vi "导轨移动.vi"(0 "绝对位置":dbl, 1 "速度":i32, 5 "高温平板相对位置":dbl, 7 "低温平板相对位置":dbl, 11 "error in":errorcluster, 12 "移动至高温？":bool, 13 "默认位置":bool, 14 "执行程序零":bool) -> (8 "位置坐标":dbl, 15 "error IO":errorcluster)   [LabVIEW 2016]
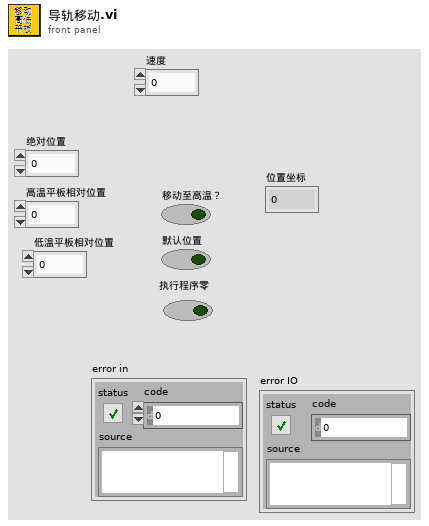
[diagram p1: front panel]
types:
  T1 = enum16{"read", "write", "release", "initial", "position calibration"}
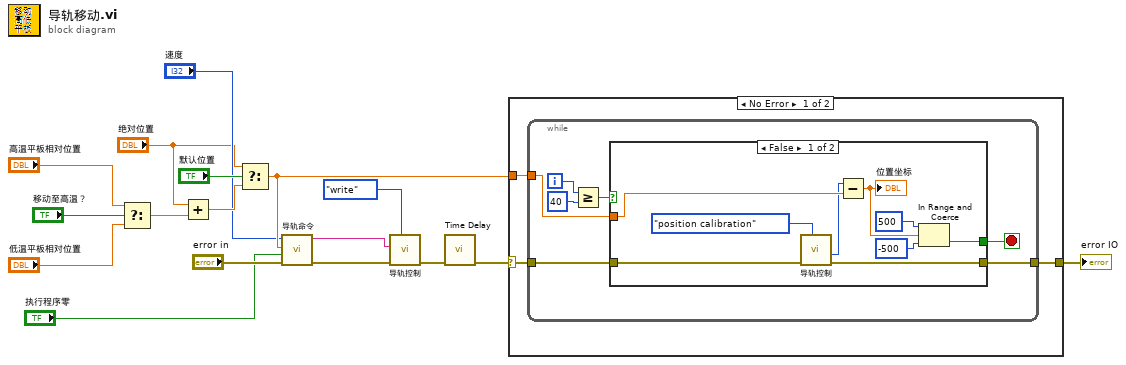
[diagram p0: block diagram]
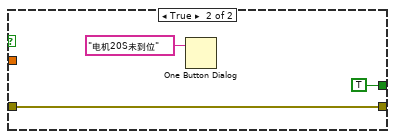
[diagram p2: hidden frame]
diagram:
  n1 = Select(t="高温平板相对位置", s="移动至高温？", f="低温平板相对位置") -> (s? t:f=w12:dbl)
  n2 = Add(x="绝对位置", y=w12) -> (x+y=w11:dbl)
  n3 = Select(t="绝对位置", s="默认位置", f=w11) -> (s? t:f=w5:dbl)
  n4 = call "导轨命令.vi"("error in"="error in", "执行程序零"="执行程序零", "绝对位置"=w5, "速度"="速度") -> ("error out"=w17:errorcluster, "输出字符串"=w16:string)  [unwired: 6 in]
  n5 = call "导轨控制.vi"("Enum"=T1."write", "error in"=w17, "write buffer"=w16) -> ("error out"=w8:errorcluster)  [unwired: 6 in, 2 out]
  n6 = call "Time Delay"("error in (no error)"=w8) -> ("error out"=w7:errorcluster)  [unwired: 10 in]
  n7 = case shown="No Error" w7 {
    selector: w7 -> [w20 w40]
    tunnel: [w19 w40] -> w9
    tunnel: w5 -> [w18 _]
    frame No Error {
      n8 = while {
        tunnel: w20 -> [w25]
        tunnel: [w24] -> w19
        tunnel: w18 -> [w23]
        i -> [w26]
        stop <- w22 stop-if-true
        n9 = Greater Or Equal?(x=w26, y=40) -> (x >= y?=w21:bool)
        n10 = case shown="False" w21 {
          tunnel: w25 -> [w35 w39]
          tunnel: [w34 w39] -> w24
          tunnel: w23 -> [w30 _]
          tunnel: [w28 TRUE] -> w22
          frame False {
            n11 = call "导轨控制.vi"("Enum"=T1."position calibration", "error in"=w35) -> ("error out"=w34:errorcluster, "position"=w29:i32)  [unwired: 7 in, 1 out]
            n12 = Subtract(x=w29, y=w30) -> (x-y=w33:dbl)
            "位置坐标" <- w33
            n13 = In Range and Coerce(upper limit=500, x=w33, lower limit=-500) -> (In Range?=w28:bool)  [unwired: 1 out]
          }
          frame True {
            n14 = One Button Dialog(message="电机20S未到位") -> ()  [unwired: 1 in, 1 out]
          }
        }
      }
    }
    frame Error {
    }
  }
  "error IO" <- w9
